vi "Read Aout Point.vi"(8 "error in (no error)":errorcluster, 11 "VISA resource name":refnum<visa-resource-name>) -> (0 "error out":errorcluster, 2 "aout point":cluster{"APointC":dbl, "APointL":dbl}={"APointC"=20.0, "APointL"=20.0}, 3 "VISA resource name out":refnum<visa-resource-name>)   [LabVIEW 2024, in "Andeen-Hagerling 2700A.lvlib"]
doc: "Returns the value of the analog out setpoint parameter."
uses:
  Andeen-Hagerling 2700A.lvlib
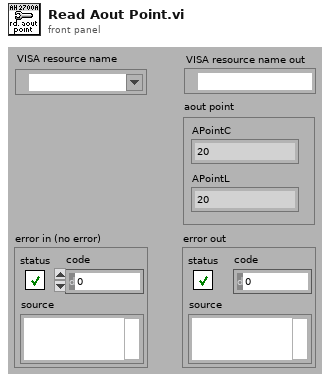
[diagram p1: front panel]
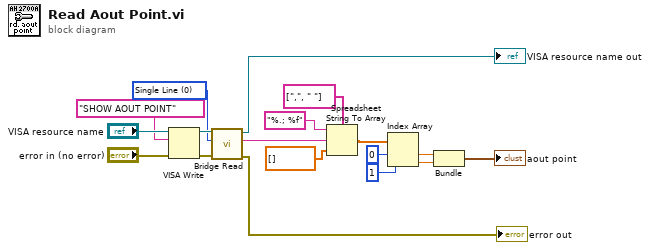
[diagram p0: block diagram]
diagram:
  w1 = u16 0 items=["Single Line", "Multi-Line"] ("Multiline")
  n1 = VISA Write(VISA resource name="VISA resource name", write buffer="SHOW AOUT POINT" ("command"), error in (no error)="error in (no error)") -> (VISA resource name out=w13:refnum<visa-resource-name>, error out=w12:errorcluster)  [unwired: 1 out]
  n2 = call "Bridge Read.vi"("error in (no error)"=w12, "multiline"=w1, "VISA resource name"=w13) -> ("error out"=→"error out":errorcluster, "read buffer"=w10:string, "VISA resource name out"=→"VISA resource name out":refnum<visa-resource-name>)  [unwired: 6 in]
  n3 = Spreadsheet String To Array(delimiter (Tab)=string[] [",", " "], format string="%.; %f", spreadsheet string=w10, array type (2D Dbl)=dbl[] []) -> (array=w3:dbl[])
  n4 = Index Array(array=w3, index #1=0 ("index"), index #2=1 ("index")) -> (element #1=w5:dbl, element #2=w4:dbl)
  n5 = Bundle(w5, w4) -> (→"aout point":cluster{dbl, dbl})  [unwired: 1 in]
